vi "Read Motor Position.vi"(8 "error in (no error)":errorcluster, 10 "Motor ID (0)":u8, 11 "VISA resource name":refnum<visa-resource-name>) -> (0 "error out":errorcluster, 2 "Position (deg)":dbl, 3 "VISA resource name out":refnum<visa-resource-name>)   [LabVIEW 2016, in "Dynamixel Motor.lvlib"]
doc: "Reads the motor's position."
uses:
  Dynamixel Motor.lvlib
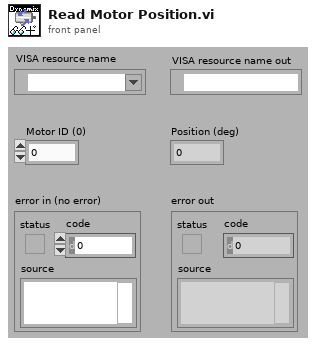
[diagram p1: front panel]
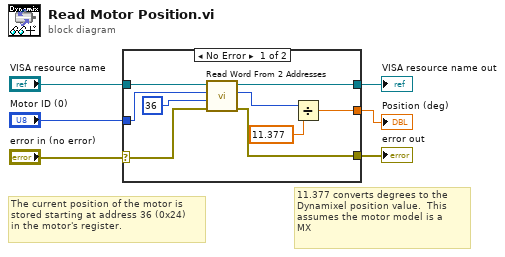
[diagram p0: block diagram]
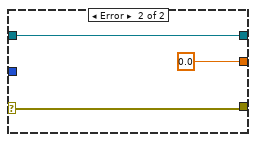
[diagram p2: hidden frame]
diagram:
  # "The current position of the motor is\nstored starting at address 36 (0x24)\nin the motor's register."
  # "11.377 converts degrees to the \nDynamixel position value.  This \nassumes the motor model is a \nMX"
  n1 = case shown="No Error" "error in (no error)" {
    selector: "error in (no error)" -> [w7 w17]
    tunnel: "VISA resource name" -> [w15 w18]
    tunnel: [w14 w18] -> w5
    tunnel: [w13 w17] -> w4
    tunnel: [w10 0.0] -> w3
    tunnel: "Motor ID (0)" -> [w9 _]
    frame No Error {
      n2 = call "Read Word From 2 Addresses.vi"("Error in (no error)"=w7, "Address number (0)"=u8 36 ("Address # DEC"), "Motor ID (0)"=w9, "VISA resource name"=w15) -> ("error out"=w13:errorcluster, "Data"=w12:u16, "VISA resource name out"=w14:refnum<visa-resource-name>)  [unwired: 5 in]
      n3 = Divide(x=w12, y=11.377) -> (x/y=w10:dbl)
    }
    frame Error {
    }
  }
  "VISA resource name out" <- w5
  "error out" <- w4
  "Position (deg)" <- w3
